vi "ATE-CalPopup.vi"(4 "Second Button Name":string="Cancel", 5 "Show 'Cancel' Button":bool=TRUE, 6 "Button Name":string="OK", 8 "error in (no error)":errorcluster, 9 "Enable":bool=TRUE, 10 "Message":string) -> (0 "error out":errorcluster, 2 "OK":bool)   [LabVIEW 2018]
doc: "Displays a standard dialog box that contains an alert or a message for users."
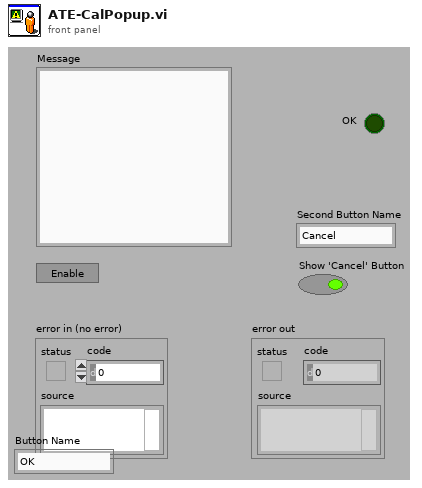
[diagram p1: front panel]
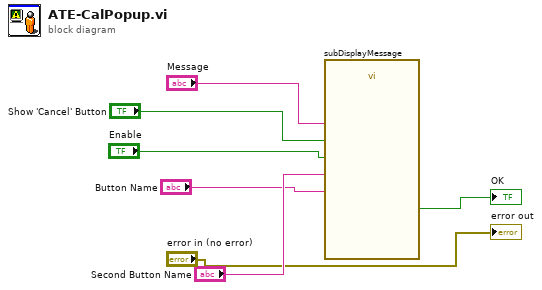
[diagram p0: block diagram]
diagram:
  n1 = call <vilib>:"subDisplayMessage.vi"("Second Button Name"="Second Button Name", "Button Name"="Button Name", "Enable Message"="Enable", "Show 'Cancel' Button"="Show 'Cancel' Button", "Message to Display"="Message") -> ("OK?"=→"OK":bool)  [unwired: 5 in, 1 out]
  "error out" <- "error in (no error)"
